vi "Register for Broadcast Events.vi"(8 "error in (no error)":errorcluster, 11 "Helper Loop in":refnum<class "Helper Loop.lvclass">) -> (0 "error out":errorcluster, 2 "Event Registration Refnum":refnum<event-registration>, 3 "Helper Loop out":refnum<class "Helper Loop.lvclass">)   [LabVIEW 2020, in "Helper Loop.lvclass"]
uses:
  Helper Loop.lvclass
  Process/Protected/Broadcasting/Broadcast Message Cluster.ctl
  Process/Process.lvclass
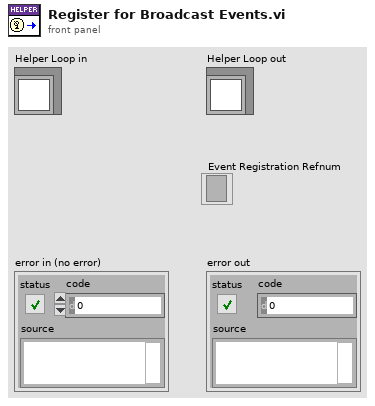
[diagram p1: front panel]
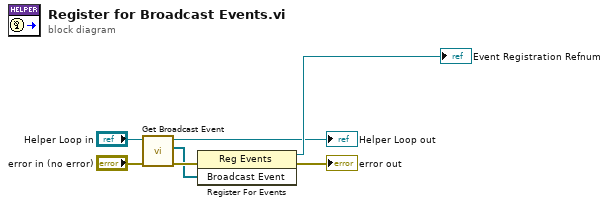
[diagram p0: block diagram]
diagram:
  n1 = call-dynamic "Get Broadcast Event.vi"("error in (no error)"="error in (no error)", "Helper Loop in"="Helper Loop in") -> ("error out"=w5:errorcluster, "Broadcast Event"=w4:refnum<user-event>[], "Helper Loop out"=→"Helper Loop out":refnum<class "Helper Loop.lvclass">)  [unwired: 7 in]
  n2 = register-events(error in=w5, w4) -> (reference out=→"Event Registration Refnum":refnum<event-registration>, error out=→"error out":errorcluster)  [unwired: 1 in]
